vi "Class_Find Match in Array.vi"(6 "Groups To Find":refnum<class>, 7 "GroupList":refnum<class>[](array[class])) -> (2 "Index Of Element Out":i32, 3 "(Group).lvclass Out":refnum<class>)   [LabVIEW 2020]
uses:
  error/Error Eater.vi
  <vilib>/Utility/LVClass/Get LV Class Name.vi
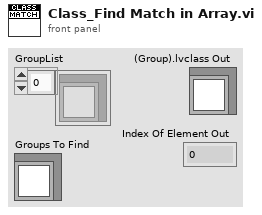
[diagram p1: front panel]
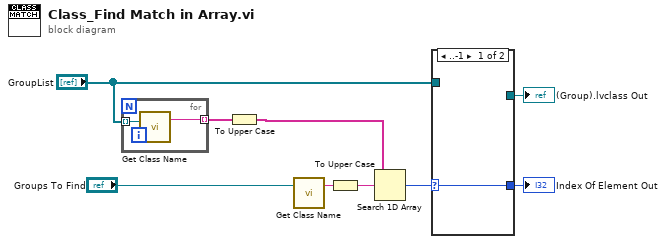
[diagram p0: block diagram]
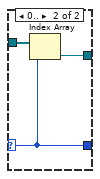
[diagram p2: hidden frame]
diagram:
  n1 = for {
    tunnel: "GroupList" -> [w11] mode=indexing
    tunnel: [w10] -> w9 mode=indexing
    n2 = call "Get Class Name.vi"("lvclass"=w11) -> ("Child Name"=w10:string)  [unwired: 3 in, 1 out]
  }
  n3 = To Upper Case(1:w9) -> (0:w8:string[])
  n4 = call "Get Class Name.vi"("lvclass"="Groups To Find") -> ("Child Name"=w6:string)  [unwired: 3 in, 1 out]
  n5 = To Upper Case(1:w6) -> (0:w5:string)
  n6 = Search 1D Array(1D array=w8, element=w5) -> (index of element=w4:i32)  [unwired: 1 in]
  n7 = case shown="..-1" w4 {
    selector: w4 -> [w12 w13]
    tunnel: "GroupList" -> [_ w15]
    tunnel: [_ w14] -> w2
    tunnel: [w12 w13] -> w1
    frame ..-1 {
    }
    frame 0.. {
      n8 = Index Array(array=w15, index=w13) -> (element=w14:refnum<class>)
    }
  }
  "(Group).lvclass Out" <- w2
  "Index Of Element Out" <- w1
